vi "649SetFinalAppTool.vi"() -> (7 "Out Arr":string[][](array[string]), 8 "?":string[](array[string]), 10 "Boolean":bool)   [LabVIEW 2023]
uses:
  <vilib>/numeric/Random Number (Range) U64.vi
  <vilib>/numeric/sub_Random U32.vi
  <vilib>/Utility/file.llb/Write Delimited Spreadsheet (string).vi
panel:
  out "Final Array":string[][](array[string])
  out "error out 2":errorcluster
  out "error out":errorcluster
  in  "?":bool
  # "6@49"
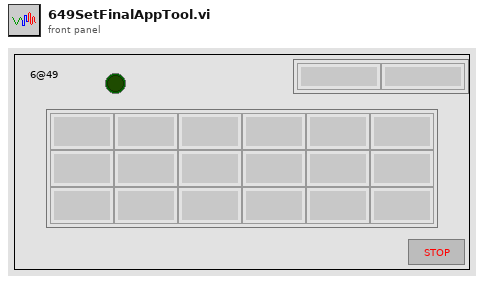
[diagram p1: front panel]
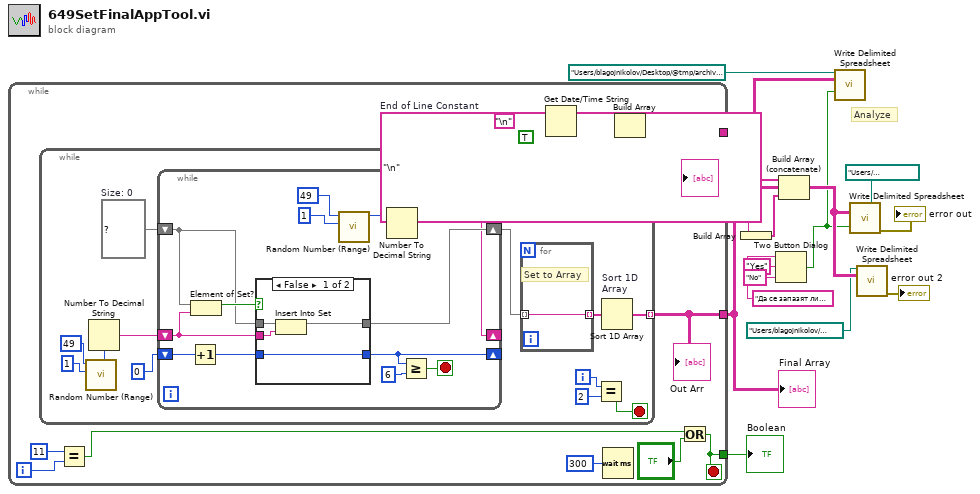
[diagram p0: block diagram]
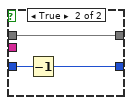
[diagram p2: hidden frame]
diagram:
  w12 = "\n"  # End of Line Constant
  # "Analyze"
  n1 = while {
    tunnel: [w27] -> w11
    tunnel: [w22] -> w15
    tunnel: [w16] -> w3
    i -> [w19]
    stop <- w16 stop-if-true
    n2 = while {
      tunnel: [w28] -> w27 mode=indexing
      i -> [w34]
      stop <- w32 stop-if-true
      w39 = set{string} {}  # Size: 0
      n3 = call-poly <vilib>:"Random Number (Range).vi"("lower bound (0)"=u64 1, "upper bound (100)"=u64 49) -> ("number"=w36:u64)  [unwired: 9 in]
      n4 = Number To Decimal String(number=w36) -> (decimal integer string=w35:string)  [unwired: 1 in]
      n5 = while {
        shift-right: [w44] -> _
        shift-left: w35 -> [w45]
        shift-right: [w51] -> w30
        shift-left: w39 -> [w52]
        shift-right: [w43] -> _
        shift-left: 0 -> [w42]
        stop <- w50 stop-if-true
        n6 = Increment(x=w42) -> (x+1=w41:i32)
        n7 = Element of Set?(10:w45, 11:w52) -> (3:w53:bool)
        n8 = case shown="False" w53 {
          tunnel: w52 -> [w57 w60]
          tunnel: [w56 w60] -> w51
          tunnel: w41 -> [w55 w59]
          tunnel: [w55 w58] -> w43
          tunnel: w45 -> [w54 _]
          frame False {
            n9 = Insert Into Set(10:w54, 11:w57) -> (3:w56:set{string})  [unwired: 1 out]
          }
          frame True {
            n10 = Decrement(x=w59) -> (x-1=w58:i32)
          }
        }
        n11 = call-poly <vilib>:"Random Number (Range).vi"("lower bound (0)"=u64 1, "upper bound (100)"=u64 49) -> ("number"=w46:u64)  [unwired: 9 in]
        n12 = Number To Decimal String(number=w46) -> (decimal integer string=w44:string)  [unwired: 1 in]
        n13 = Greater Or Equal?(x=w43, y=6) -> (x >= y?=w50:bool)
      }
      n14 = for {
        tunnel: [w40] -> w29 mode=indexing
        tunnel: w30 -> [w40] mode=indexing
        # "Set to Array"
      }
      n15 = Equal?(x=w34, y=2) -> (x = y?=w32:bool)
      n16 = Sort 1D Array "Sort 1D \nArray"(array=w29) -> (sorted array=w28:string[])
    }
    "Out Arr" <- w27
    n17 = Equal?(x=11, y=w19) -> (x = y?=w17:bool)
    n18 = Get Date/Time String(want seconds? (F)=TRUE) -> (date string=w24:string, time string=w25:string)  [unwired: 2 in]
    n19 = Wait (ms)(milliseconds to wait=u32 300) -> ()  [unwired: 1 out]
    n20 = Build Array(w24, w25, "\n") -> (w22:string[])
    "?" <- w22
    n21 = Or(x=w17, y="?") -> (x .or. y?=w16:bool)
  }
  "Final Array" <- w11
  "Boolean" <- w3
  n22 = Build Array(w12) -> (w14:string[])
  n23 = Two Button Dialog(message="Да се запазят ли предишните резултати ?", 1:"No" ("F button name (\"Cancel\")"), 2:"Yes" ("T button name (\"OK\")")) -> (T button?=w4:bool)
  n24 = Build Array (concatenate) "Build Array"(w15, w11, w14) -> (w7:string[][])
  n25 = call-poly <vilib>:"Write Delimited Spreadsheet.vi"("file path (dialog if empty)"=path "/Users/blagojnikolov/Desktop/@tmp/archive.txt", "2D data"=w11, "append to file? (new file:F)"=w4) -> ()  [unwired: 11 in, 2 out]
  n26 = call-poly <vilib>:"Write Delimited Spreadsheet.vi"("file path (dialog if empty)"=path "/Users/blagojnikolov/Desktop/@tmp/toto.txt", "2D data"=w7, "append to file? (new file:F)"=w4) -> ("error out"=→"error out":errorcluster)  [unwired: 11 in, 1 out]
  n27 = call-poly <vilib>:"Write Delimited Spreadsheet.vi"("file path (dialog if empty)"=path "/Users/blagojnikolov/Desktop/@tmp/checkRes.txt", "2D data"=w7) -> ("error out"=→"error out 2":errorcluster)  [unwired: 12 in, 1 out]
